vi "Arduino_Comms.vi"() -> ()   [LabVIEW 2012]
uses:
  <vilib>/Instr/_visa.llb/VISA Configure Serial Port (Instr).vi
panel:
  out "Waveform Chart":i32(graph)
  in  "Set Point":u8
  in  "Write":bool
  out "Response":string
  in  "stop":bool
  in  "Arduino Port":refnum<visa-resource-name>="COM8"
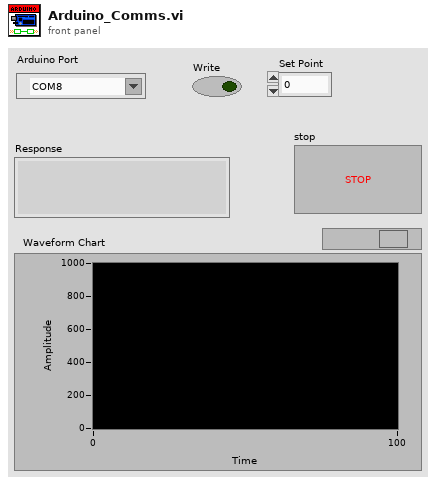
[diagram p1: front panel]
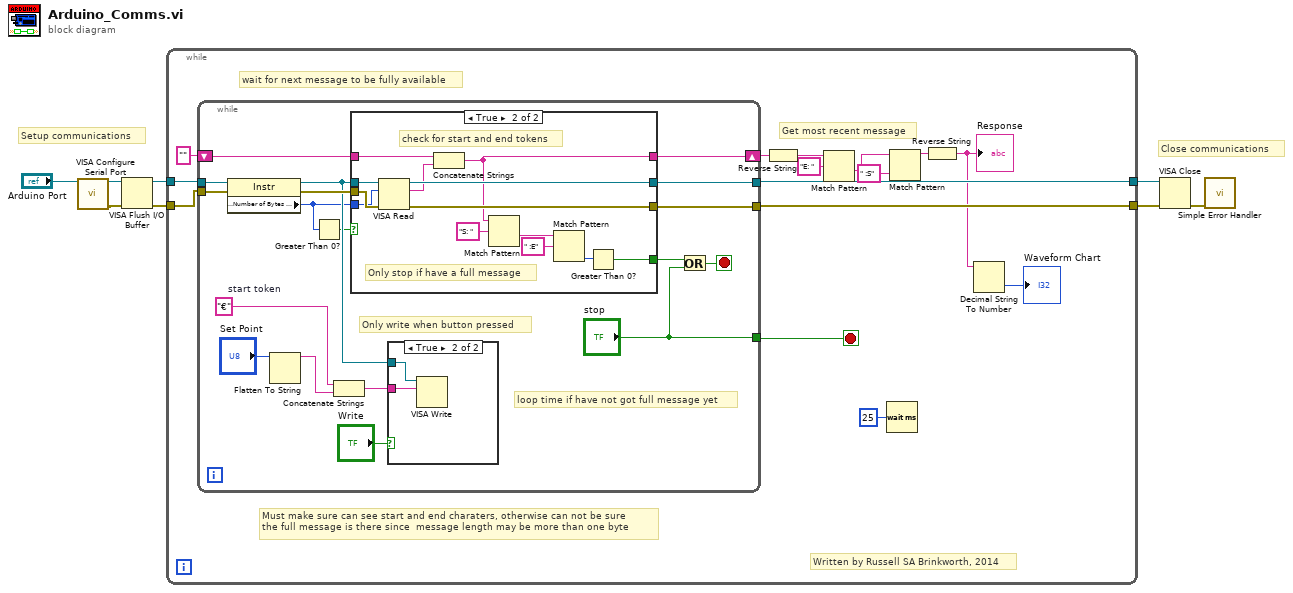
[diagram p0: block diagram]
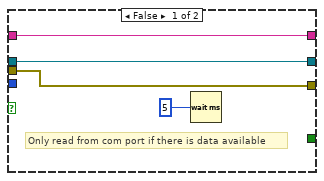
[diagram p3: hidden frame]
diagram:
  # "Close communications"
  # "Setup communications"
  n1 = call-poly "VISA Configure Serial Port"("VISA resource name"="Arduino Port") -> ("VISA resource name out"=w3:refnum<visa-resource-name>, "error out"=w4:errorcluster)  [unwired: 8 in, 5 out]
  n2 = VISA Flush I/O Buffer(VISA resource name=w3, error in (no error)=w4) -> (VISA resource name out=w1:refnum<visa-resource-name>, error out=w2:errorcluster)  [unwired: 1 in]
  n3 = while {
    tunnel: w1 -> [w17]
    tunnel: w2 -> [w22]
    tunnel: [w21] -> w6
    tunnel: [w20] -> w7
    stop <- w18 stop-if-true
    # "Written by Russell SA Brinkworth, 2014"
    # "Get most recent message"
    # "Must make sure can see start and end charaters, otherwise can not be sure \nthe full message is there since  message length may be more than one byte"
    # "wait for next message to be fully available"
    n4 = while {
      tunnel: w17 -> [w41]
      tunnel: w22 -> [w40]
      tunnel: [w38] -> w21
      tunnel: [w37] -> w20
      shift-right: [w36] -> w10
      shift-left: "" -> [w35]
      tunnel: ["stop"] -> w18
      stop <- w33 stop-if-true
      w26 = "€"  # start token
      # "loop time if have not got full message yet"
      # "Only write when button pressed"
      n5 = property class="Instr"(reference=w41, error in=w40) -> (reference out=w31:refnum<visa-resource-name>, error out=w39:errorcluster, "Serial Settings:Number of Bytes at Serial Port"=w24:u32)
      n6 = Flatten To String(anything="Set Point") -> (data string=w28:string)  [unwired: 3 in, 2 out]
      n7 = Greater Than 0?(x=w24) -> (x > 0?=w25:bool)
      n8 = Concatenate Strings(w26, w28) -> (w27:string)
      n9 = case shown="True" w25 {
        tunnel: w24 -> [_ w58]
        tunnel: w31 -> [w47 w60]
        tunnel: w39 -> [w46 w59]
        tunnel: [w47 w57] -> w38
        tunnel: [w46 w56] -> w37
        tunnel: [_ w55] -> w34
        tunnel: w35 -> [w45 w51]
        tunnel: [w45 w50] -> w36
        frame False {
          # "Only read from com port if there is data available"
          n10 = Wait (ms)(milliseconds to wait=u32 5) -> ()  [unwired: 1 out]
        }
        frame True {
          # "check for start and end tokens"
          # "Only stop if have a full message"
          n11 = VISA Read(VISA resource name=w60, byte count=w58, error in (no error)=w59) -> (VISA resource name out=w57:refnum<visa-resource-name>, read buffer=w52:string, error out=w56:errorcluster)  [unwired: 1 out]
          n12 = Concatenate Strings(w51, w52) -> (w50:string)
          n13 = Match Pattern(string=w50, regular expression="S: ") -> (after substring=w53:string)  [unwired: 1 in, 3 out]
          n14 = Match Pattern(string=w53, regular expression=" :E") -> (offset past match=w54:i32)  [unwired: 1 in, 3 out]
          n15 = Greater Than 0?(x=w54) -> (x > 0?=w55:bool)
        }
      }
      n16 = case shown="True" "Write" {
        tunnel: w31 -> [_ w43]
        tunnel: w27 -> [_ w42]
        frame False {
        }
        frame True {
          n17 = VISA Write(VISA resource name=w43, write buffer=w42) -> ()  [unwired: 1 in, 3 out]
        }
      }
      n18 = Or(x=w34, y="stop") -> (x .or. y?=w33:bool)
    }
    n19 = Reverse String(1:w10) -> (0:w15:string)
    n20 = Match Pattern(string=w15, regular expression="E: ") -> (after substring=w11:string)  [unwired: 1 in, 3 out]
    n21 = Wait (ms)(milliseconds to wait=u32 25) -> ()  [unwired: 1 out]
    n22 = Match Pattern(string=w11, regular expression=" :S") -> (before substring=w12:string)  [unwired: 1 in, 3 out]
    n23 = Reverse String(1:w12) -> (0:w9:string)
    "Response" <- w9
    n24 = Decimal String To Number(string=w9) -> (number=→"Waveform Chart":i32)  [unwired: 2 in, 1 out]
  }
  n25 = VISA Close(VISA resource name=w6, error in (no error)=w7) -> (error out=w5:errorcluster)
  n26 = call <vilib>:"Simple Error Handler.vi"("error in (no error)"=w5) -> ()  [unwired: 1 in, 8 out]
